vi "DisableShoot.vi"(8 "error in (no error)":errorcluster, 10 "On For (0 = Forever)":dbl) -> (0 "error out":errorcluster)   [LabVIEW 2015]
uses:
  Solenoids/Solenoids.ctl
  <vilib>/Rock Robotics/WPI/Solenoid/WPI_SolenoidValue.ctl
  <vilib>/Rock Robotics/Network Tables/NT Write Boolean.vi
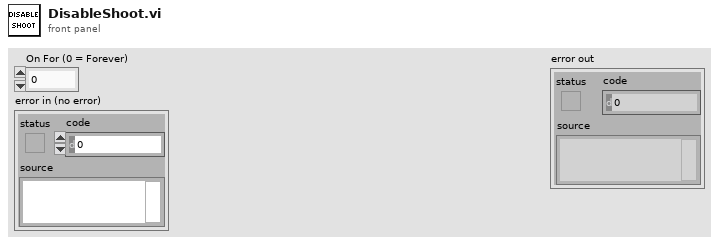
[diagram p1: front panel]
types:
  T1 = typedef "WPI_SolenoidValue.ctl" = enum16{"Off", "On", "Forward", "Reverse"}
  T2 = typedef "Solenoids.ctl" = enum16{"Gear Low", "Gear High", "Shoot Ball", "Hold Ball", "PTO Active", "PTO De-Active"}
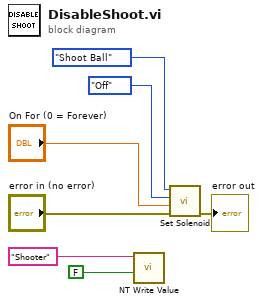
[diagram p0: block diagram]
diagram:
  n1 = call-poly <vilib>:"NT Write Value.vi"("Boolean"=FALSE, "Name"="Shooter") -> ()  [unwired: 9 in, 1 out]
  n2 = call "Set Solenoid.vi"("error in (no error)"="error in (no error)", "On For (0 = Forever)"="On For (0 = Forever)", "Value"=WPI_SolenoidValue."Off", "Solenoids"=Solenoids."Shoot Ball") -> ("error out"=→"error out":errorcluster)  [unwired: 7 in]
